vi "G#Installer.vi"() -> ()   [LabVIEW 2012, in "G#Installer.lvlib"]
uses:
  Install-support/G#Installer.lvlib
  <vilib>/Utility/error.llb/DialogType.ctl
panel:
  in  "Uninstall":bool
  out "Info":string
  in  "Cancel":bool
  out "License":string="G# Framework\n\nCopyright (c) 2010-2016, AddQ Consulting <http://www.addq.se>\n\nAll rights reserved.\n\n3-clause license (\"New BSD License\" or \"Modified BSD License\")\n(http://en.wikipedia.org/wiki/BSD_license#3-clause_license_.28.22New_BSD_License.22_or_.22Modified_BSD_License.22.29)\n--------------------------------------------------------------------\nBSD LICENSE  (http://www.opensource.org/licenses/bsd-license.php).\n\nRedistribution and use in source and binary forms, with or without modification, are permitted provided that the following conditions are met:\n\nRedistributions of source code must retain the above copyright notice, this list of conditions and the following disclaimer. Redistributions in binary form must reproduce the above copyright notice, this list of conditions and the following disclaimer in the documentation and/or other materials provided with the distribution. Neither the name of AddQ nor the names of its contributors may be used to endorse or promote products derived from this software without specific prior written permission.\n\nTHIS SOFTWARE IS PROVIDED BY THE COPYRIGHT HOLDERS AND CONTRIBUTORS \"AS IS\" AND ANY EXPRESS OR IMPLIED WARRANTIES, INCLUDING, BUT NOT LIMITED TO, THE IMPLIED WARRANTIES OF MERCHANTABILITY AND FITNESS FOR A PARTICULAR PURPOSE ARE DISCLAIMED. IN NO EVENT SHALL THE COPYRIGHT HOLDER OR CONTRIBUTORS BE LIABLE FOR ANY DIRECT, INDIRECT, INCIDENTAL, SPECIAL, EXEMPLARY, OR CONSEQUENTIAL DAMAGES (INCLUDING, BUT NOT LIMITED TO, PROCUREMENT OF SUBSTITUTE GOODS OR SERVICES; LOSS OF USE, DATA, OR PROFITS; OR BUSINESS INTERRUPTION) HOWEVER CAUSED AND ON ANY THEORY OF LIABILITY, WHETHER IN CONTRACT, STRICT LIABILITY, OR TORT (INCLUDING NEGLIGENCE OR OTHERWISE) ARISING IN ANY WAY OUT OF THE USE OF THIS SOFTWARE, EVEN IF ADVISED OF THE POSSIBILITY OF SUCH DAMAGE."
  in  "Install":bool
  # "G# Installer"
  # "1. Installs G# root classes and debugger in vi.lib/addons.\n2. Installs G# IDE in resources/AddQ/G#IDE.\n3. Installs G# examples, menues and help."
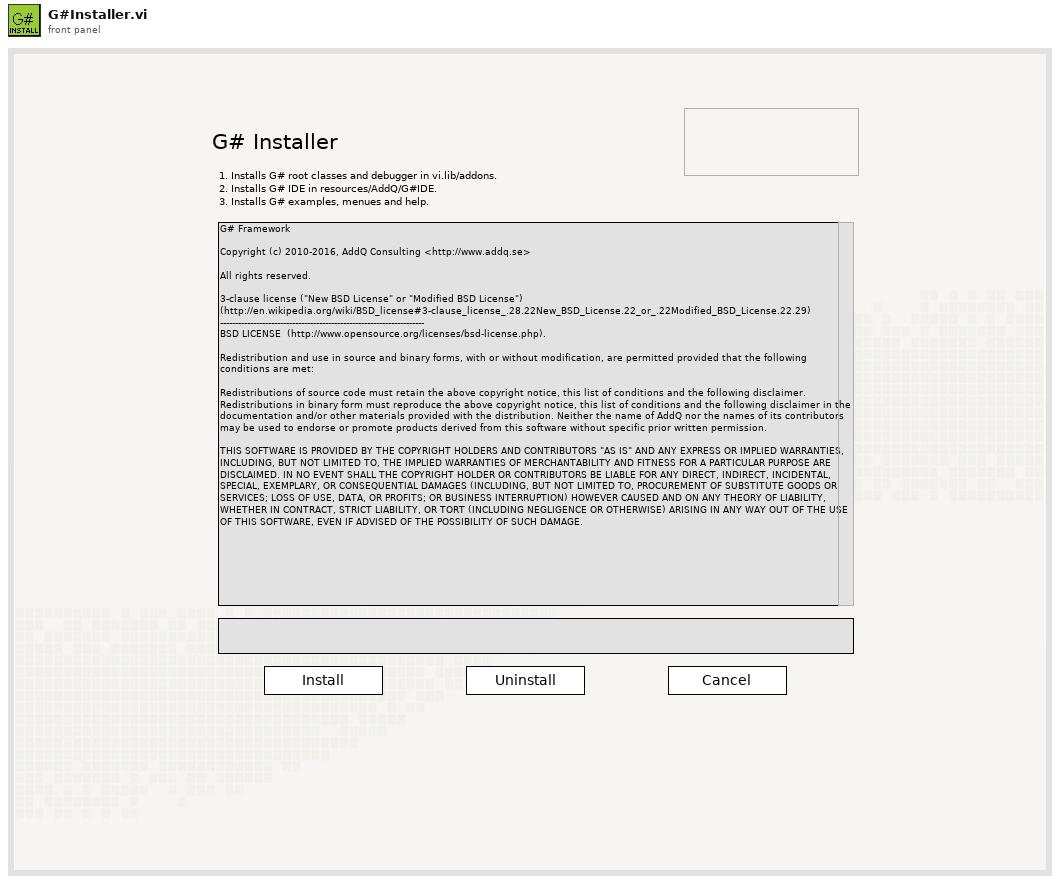
[diagram p1: front panel]
types:
  T1 = enum8{"Enabled", "Disabled", "Disabled and Grayed Out"}
  T2 = typedef "DialogType.ctl" = u16
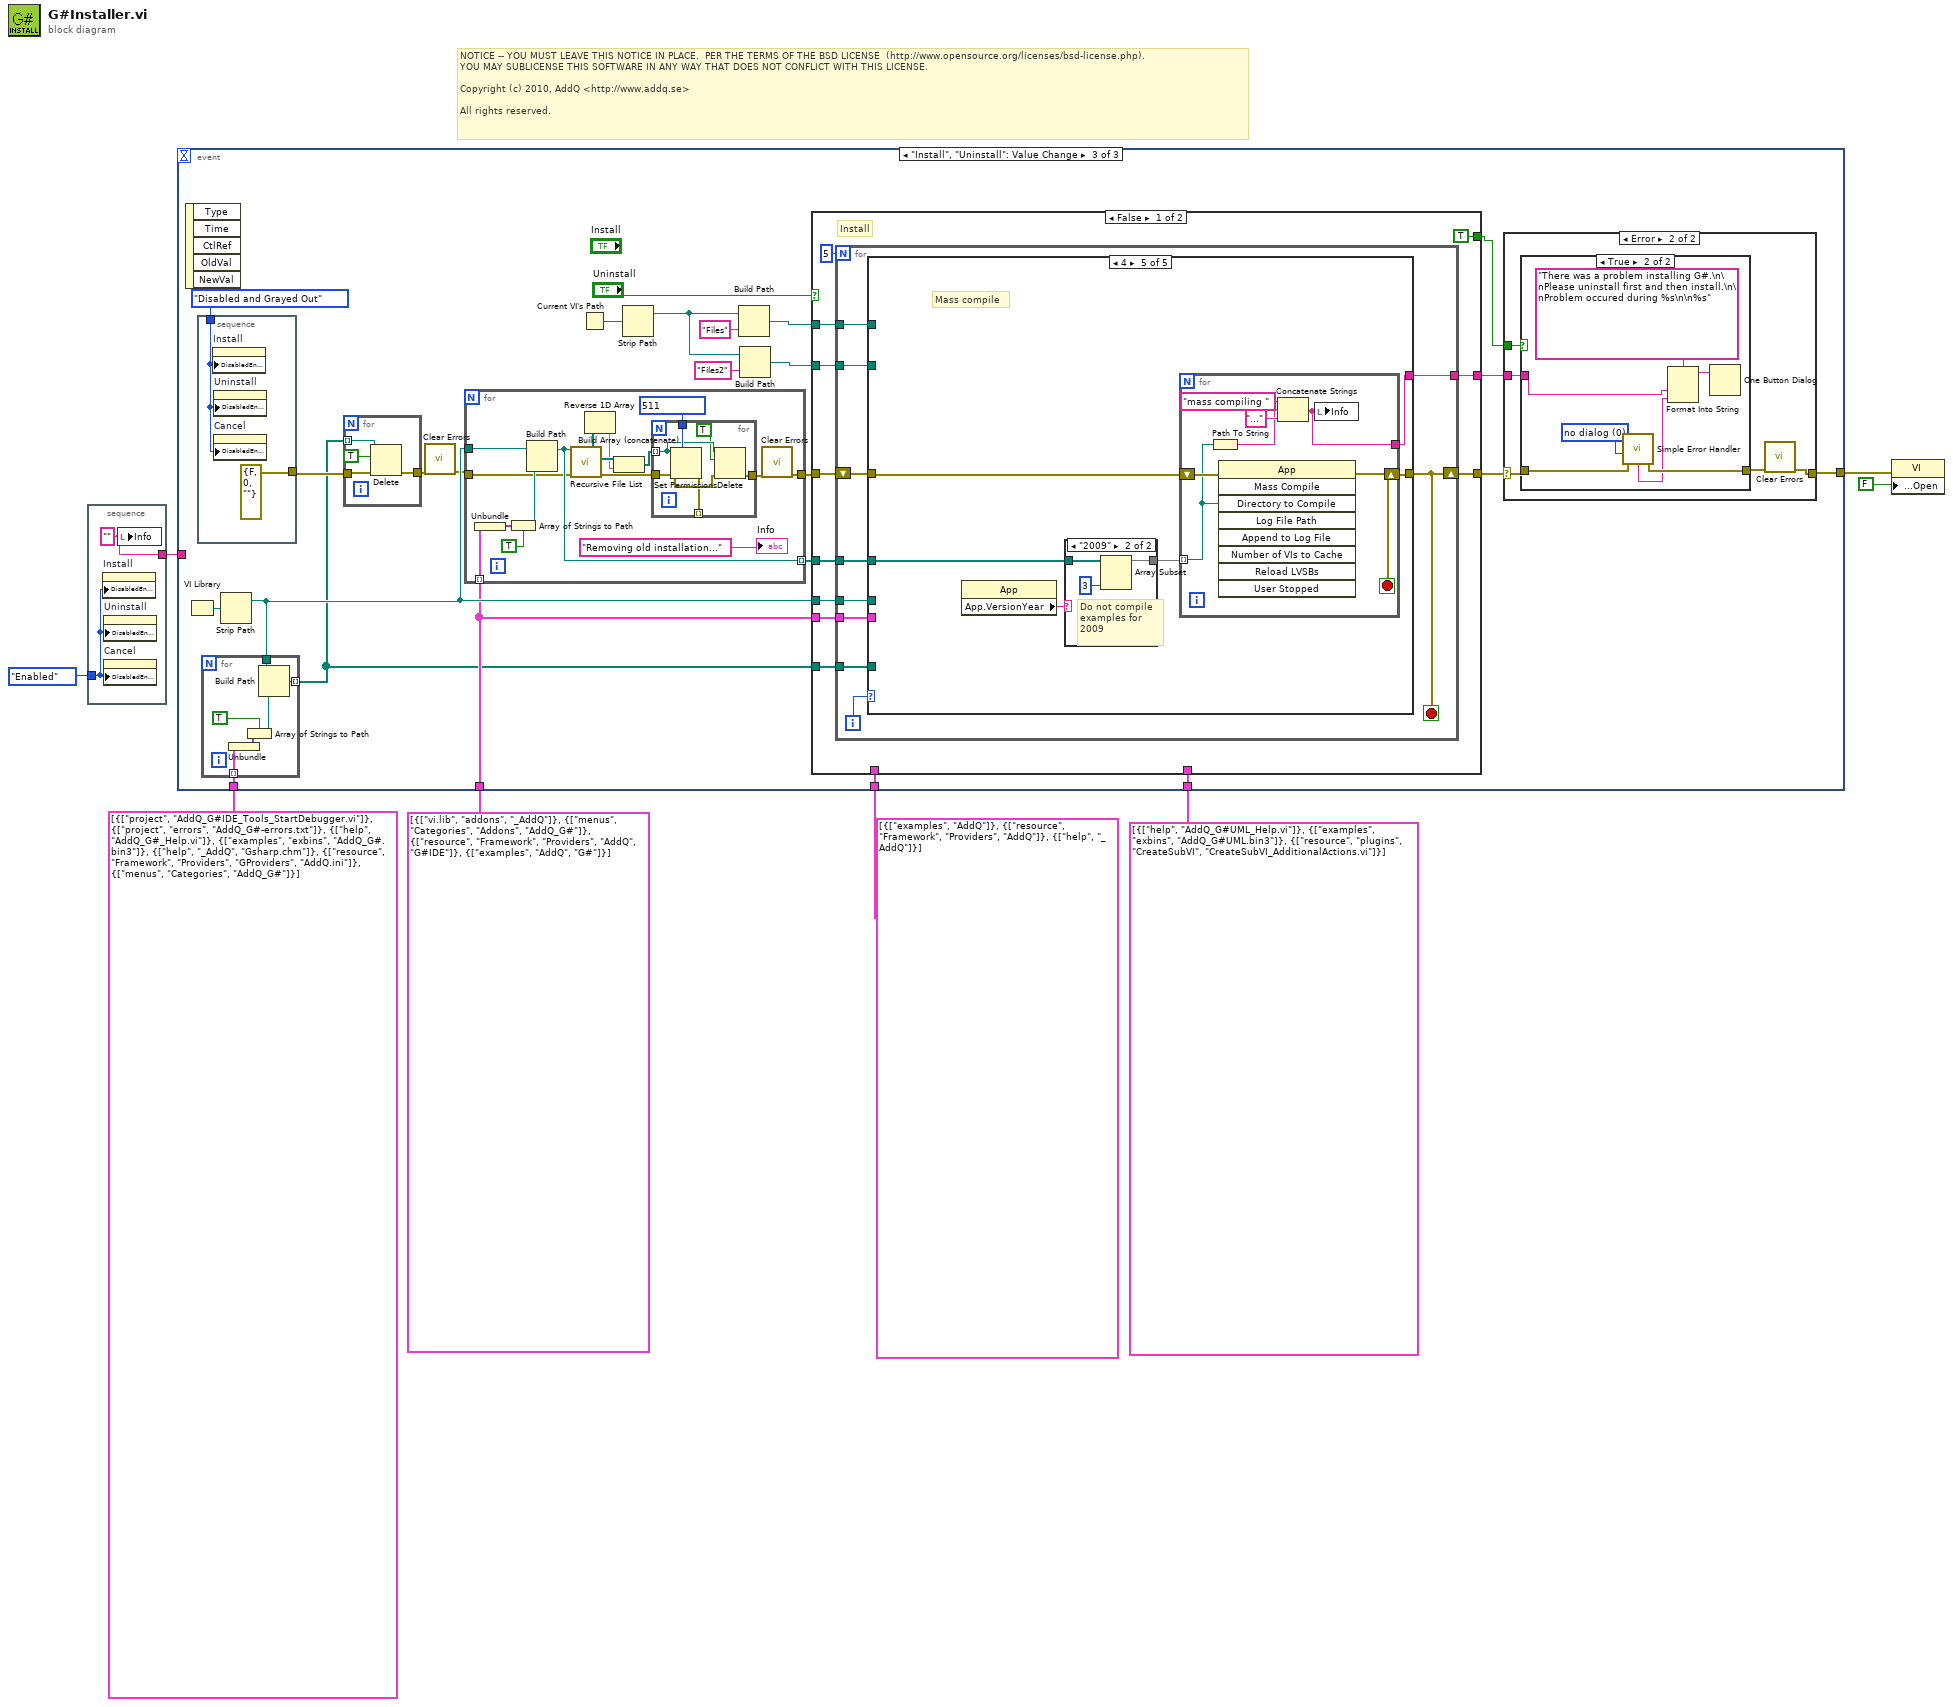
[diagram p0: block diagram]
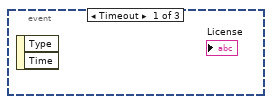
[diagram p2: hidden frame]
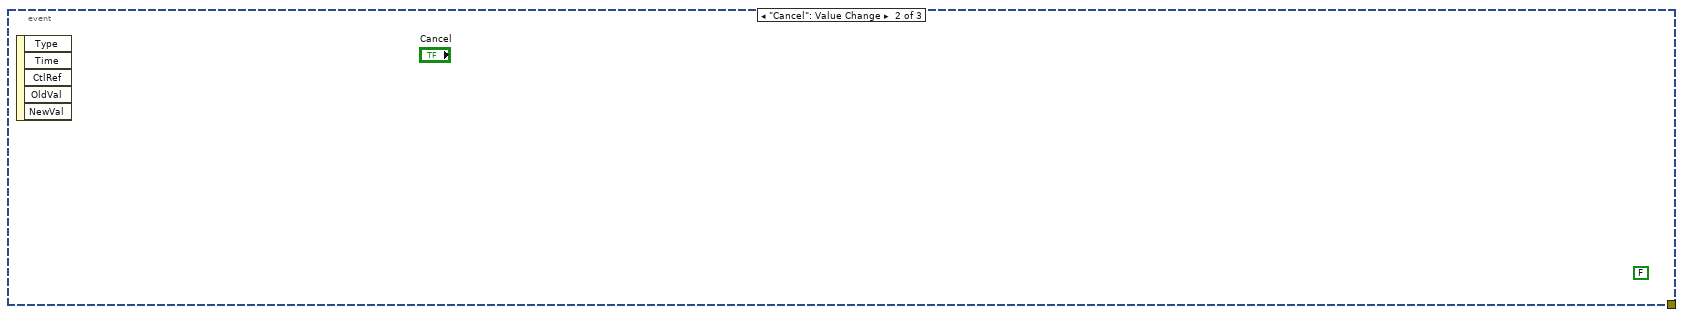
[diagram p3: hidden frame]
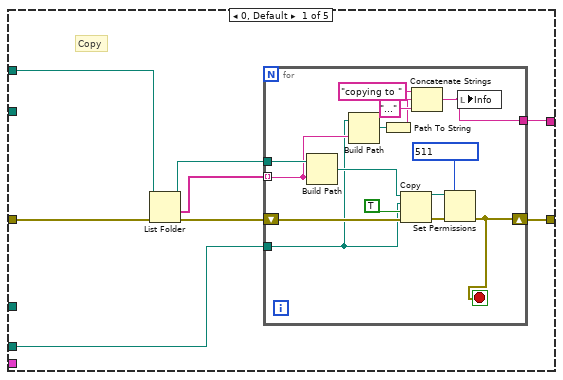
[diagram p4: hidden frame]
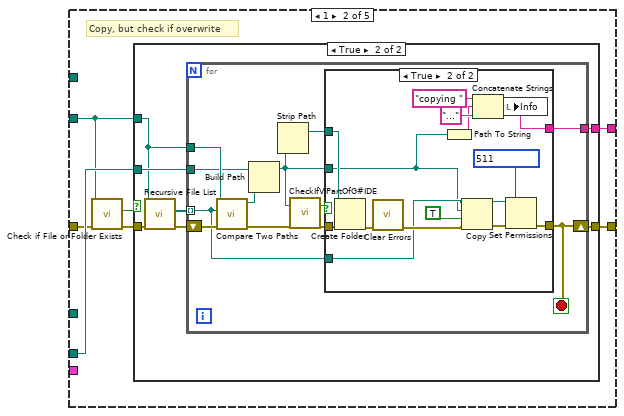
[diagram p5: hidden frame]
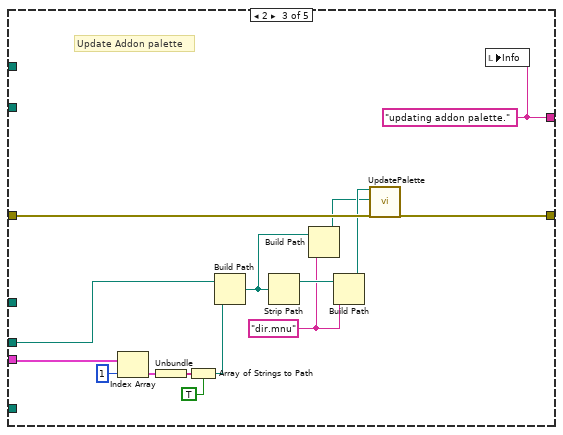
[diagram p8: hidden frame]
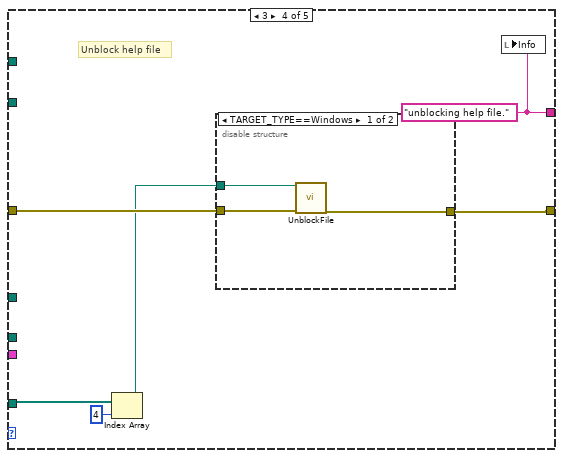
[diagram p9: hidden frame]
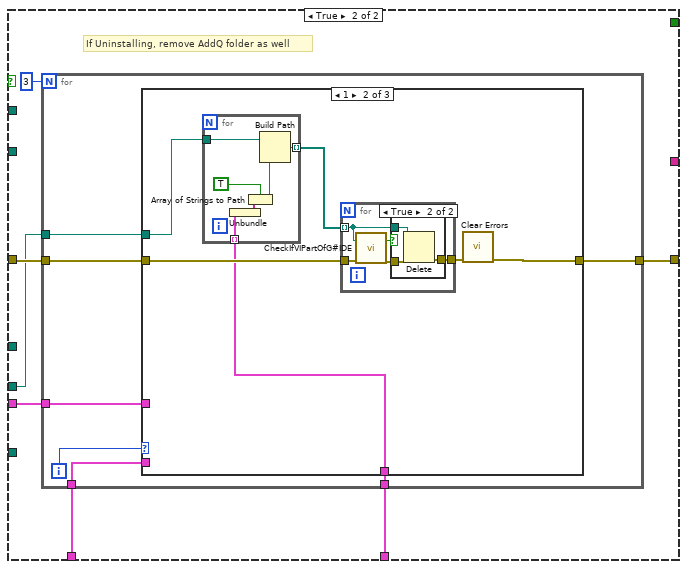
[diagram p12: hidden frame]
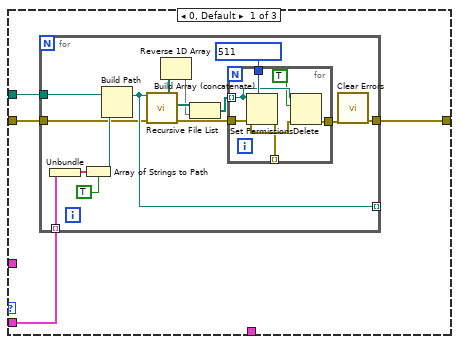
[diagram p13: hidden frame]
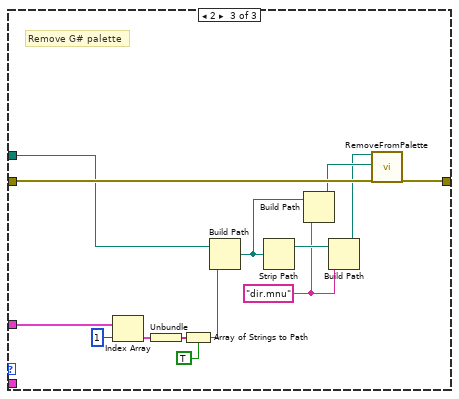
[diagram p15: hidden frame]
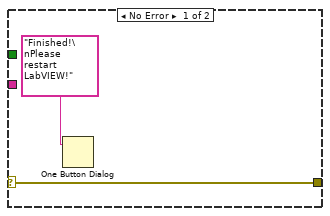
[diagram p16: hidden frame]
diagram:
  # "NOTICE -- YOU MUST LEAVE THIS NOTICE IN PLACE.  PER THE TERMS OF THE BSD LICENSE  (http://www.opensource.org/licenses/bsd-license.php).\nYOU MAY SUBLICENSE THIS SOFTWARE IN ANY WAY THAT DOES NOT CONFLICT WITH THIS LICENSE.\n\nCopyright (c) 2010, AddQ <http://www.addq.se>\n\nAll rights reserved."
  n1 = stacked-sequence {
    tunnel: [w10] -> w8
    tunnel: T1."Enabled" ("Disabled") -> [w9]
    frame #0 {
      w10 = "" ("Info")
      n2 = property on="Install" class="Bool"("DisabledEnum"=w9) -> ()  [unwired: 2 in, 2 out]
      n3 = property on="Uninstall" class="Bool"("DisabledEnum"=w9) -> ()  [unwired: 2 in, 2 out]
      n4 = property on="Cancel" class="Bool"("DisabledEnum"=w9) -> ()  [unwired: 2 in, 2 out]
      n5 = local write "Info"(w10) -> ()
    }
  }
  n6 = event shown="[2] \"Install\", \"Uninstall\": Value Change" {
    selector: _ -> [_ _ _]
    dyn-events: _ -> [_ _ _]
    timeout: _ -> [_ _ _]
    tunnel: w8 -> [_ _ _]
    tunnel: [_ _ w31] -> w1
    tunnel: cluster{string[]}[] [{["vi.lib", "addons", "_AddQ"]}, {["menus", "Categories", "Addons", "AddQ_G#"]}, {["resource", "Framework", "Providers", "AddQ", "G#IDE"]}, {["examples", "AddQ", "G#"]}] -> [_ _ w14]
    tunnel: cluster{string[]}[] [{["project", "AddQ_G#IDE_Tools_StartDebugger.vi"]}, {["project", "errors", "AddQ_G#-errors.txt"]}, {["help", "AddQ_G#_Help.vi"]}, {["examples", "exbins", "AddQ_G#.bin3"]}, {["help", "_AddQ", "Gsharp.chm"]}, {["resource", "Framework", "Providers", "GProviders", "AddQ.ini"]}, {["menus", "Categories", "AddQ_G#"]}] -> [_ _ w26]
    tunnel: cluster{string[]}[] [{["examples", "AddQ"]}, {["resource", "Framework", "Providers", "AddQ"]}, {["help", "_AddQ"]}] -> [_ _ w25]
    tunnel: cluster{string[]}[] [{["help", "AddQ_G#UML_Help.vi"]}, {["examples", "exbins", "AddQ_G#UML.bin3"]}, {["resource", "plugins", "CreateSubVI", "CreateSubVI_AdditionalActions.vi"]}] -> [_ _ w24]
    event Timeout {
      n7 = event-data() -> ()  [unwired: 1 in, 2 out]
    }
    event "Cancel": Value Change {
      (unwired) FALSE ("true")
      n8 = event-data() -> ()  [unwired: 1 in, 5 out]
    }
    event "Install", "Uninstall": Value Change {
      n9 = event-data() -> ()  [unwired: 1 in, 5 out]
      n10 = VI Library() -> (path=w32:path)
      n11 = stacked-sequence {
        tunnel: T1."Disabled and Grayed Out" ("Disabled") -> [w36]
        tunnel: [errorcluster {"status"=FALSE, "code"=0, "source"=""} ("error out")] -> w17
        frame #0 {
          n12 = property on="Install" class="Bool"("DisabledEnum"=w36) -> ()  [unwired: 2 in, 2 out]
          n13 = property on="Uninstall" class="Bool"("DisabledEnum"=w36) -> ()  [unwired: 2 in, 2 out]
          n14 = property on="Cancel" class="Bool"("DisabledEnum"=w36) -> ()  [unwired: 2 in, 2 out]
        }
      }
      n15 = Strip Path(path=w32) -> (stripped path=w22:path)  [unwired: 1 out]
      n16 = for {
        tunnel: w22 -> [w42]
        tunnel: [w41] -> w13 mode=indexing
        tunnel: w26 -> [w40] mode=indexing
        n17 = Unbundle(w40) -> (w38:string[])
        n18 = Array of Strings to Path(0:w38, 1:TRUE ("relative")) -> (2:w37:path)
        n19 = Build Path(base path=w42, name or relative path=w37) -> (appended path=w41:path)
      }
      n20 = for {
        tunnel: [w46] -> w27
        tunnel: w17 -> [w44]
        tunnel: w13 -> [w45] mode=indexing
        n21 = Delete(path (use dialog)=w45, entire hierarchy (F)=TRUE, error in=w44) -> (error out=w46:errorcluster)  [unwired: 2 in, 2 out]
      }
      n22 = call <vilib>:"Clear Errors.vi"("error in (no error)"=w27) -> ("error out"=w16:errorcluster)  [unwired: 6 in]
      n23 = for {
        tunnel: w22 -> [w264]
        tunnel: [w263] -> w15
        tunnel: [w252] -> w28 mode=indexing
        tunnel: w14 -> [w256] mode=indexing
        tunnel: w16 -> [w250]
        n24 = Unbundle(w256) -> (w255:string[])
        n25 = Array of Strings to Path(0:w255, 1:TRUE ("relative")) -> (2:w254:path)
        n26 = Build Path(base path=w264, name or relative path=w254) -> (appended path=w252:path)
        n27 = call <vilib>:"Recursive File List.vi"("error in (no error)"=w250, "Folder Path"=w252) -> ("error out"=w262:errorcluster, "All Files in Dir"=w260:path[], "All Folders"=w258:path[])  [unwired: 5 in, 2 out]
        n28 = Reverse 1D Array(array=w258) -> (reversed array=w257:path[])
        n29 = Build Array (concatenate)(w260, w257) -> (w259:path[])
        n30 = for {
          tunnel: i16 511 ("permissions") -> [w271]
          tunnel: w262 -> [w269]
          tunnel: w259 -> [w268] mode=indexing
          tunnel: [w270] -> w261
          tunnel: [w267] -> _ mode=indexing
          n31 = Set Permissions(7:w271, 8:w269, 11:w268) -> (0:w267:errorcluster)  [unwired: 2 in, 1 out]
          n32 = Delete(path (use dialog)=w268, entire hierarchy (F)=TRUE, error in=w269) -> (error out=w270:errorcluster)  [unwired: 2 in, 2 out]
        }
        n33 = call <vilib>:"Clear Errors.vi"("error in (no error)"=w261) -> ("error out"=w263:errorcluster)  [unwired: 6 in]
        "Info" <- "Removing old installation..." ("string")
      }
      n34 = Current VI's Path() -> (path=w34:path)
      n35 = Strip Path(path=w34) -> (stripped path=w21:path)  [unwired: 1 out]
      n36 = Build Path(base path=w21, name or relative path="Files") -> (appended path=w19:path)
      n37 = Build Path(base path=w21, name or relative path="Files2") -> (appended path=w18:path)
      n38 = case shown="False" "Uninstall" {
        tunnel: w19 -> [w57 _]
        tunnel: w22 -> [w56 w180]
        tunnel: [w53 w178] -> w30
        tunnel: w28 -> [w52 _]
        tunnel: w15 -> [w55 w182]
        tunnel: w25 -> [_ w181]
        tunnel: w24 -> [_ w177]
        tunnel: w18 -> [w51 _]
        tunnel: w14 -> [w50 w176]
        tunnel: w13 -> [w49 _]
        tunnel: [w48 _] -> w12
        tunnel: [TRUE ("Install") _] -> w11
        frame False {
          # "Install"
          n39 = for {
            N: 5 -> [_]
            tunnel: w57 -> [w67]
            tunnel: w56 -> [w66]
            shift-right: [w58] -> w53
            shift-left: w55 -> [w65]
            tunnel: w52 -> [w63]
            tunnel: w51 -> [w62]
            tunnel: w50 -> [w61]
            tunnel: w49 -> [w60]
            tunnel: [w59] -> w48
            i -> [w64]
            stop <- w58 stop-if-true
            n40 = case shown="4" w64 {
              tunnel: w67 -> [w75 _ _ _ _]
              tunnel: w66 -> [w74 w97 w141 _ _]
              tunnel: w65 -> [w73 w95 w148 w154 w162]
              tunnel: [w72 w96 w135 w150 w164] -> w58
              tunnel: w63 -> [_ _ _ _ w161]
              tunnel: w62 -> [_ w93 _ _ _]
              tunnel: w61 -> [_ _ w147 _ _]
              tunnel: w60 -> [_ _ _ w153 _]
              tunnel: [w68 w91 w134 w149 w159] -> w59
              frame 0, Default {
                # "Copy"
                n41 = List Folder(path=w75, error in=w73) -> (path out=w71:path, folder names=w69:string[], error out=w70:errorcluster)  [unwired: 2 in, 1 out]
                n42 = for {
                  tunnel: w74 -> [w78]
                  tunnel: w69 -> [w79] mode=indexing
                  tunnel: w71 -> [w89]
                  shift-right: [w77] -> w72
                  shift-left: w70 -> [w86]
                  tunnel: [w76] -> w68
                  stop <- w77 stop-if-true
                  n43 = Build Path(base path=w89, name or relative path=w79) -> (appended path=w82:path)
                  n44 = Build Path(base path=w78, name or relative path=w79) -> (appended path=w80:path)
                  n45 = Path To String(path=w80) -> (string=w81:string)
                  n46 = Copy(8:w86, 9:TRUE ("overwrite (F)"), 10:w78, 11:w82) -> (0:w85:errorcluster, 3:w84:path)  [unwired: 1 in, 1 out]
                  n47 = Concatenate Strings("copying to " ("string"), w81, "..." ("string")) -> (w76:string)
                  n48 = Set Permissions(7:i16 511 ("permissions"), 8:w85, 11:w84) -> (0:w77:errorcluster)  [unwired: 2 in, 1 out]
                  n49 = local write "Info"(w76) -> ()
                }
              }
              frame 1 {
                # "Copy, but check if overwrite"
                n50 = call <vilib>:"Check if File or Folder Exists.vi"("error in (no error)"=w95, "path"=w93) -> ("error out"=w94:errorcluster, "file or folder exists?"=w92:bool)  [unwired: 7 in, 1 out]
                n51 = case shown="True" w92 {
                  tunnel: w97 -> [_ w105]
                  tunnel: [w98 w104] -> w96
                  tunnel: w94 -> [w98 w101]
                  tunnel: w93 -> [_ w100]
                  tunnel: [_ w99] -> w91
                  frame False {
                  }
                  frame True {
                    n52 = call <vilib>:"Recursive File List.vi"("error in (no error)"=w101, "Folder Path"=w100) -> ("error out"=w103:errorcluster, "All Files in Dir"=w102:path[])  [unwired: 5 in, 3 out]
                    n53 = for {
                      tunnel: w105 -> [w112]
                      tunnel: w102 -> [w108] mode=indexing
                      shift-right: [w106] -> w104
                      shift-left: w103 -> [w116]
                      tunnel: w100 -> [w114]
                      tunnel: [w107] -> w99
                      stop <- w106 stop-if-true
                      n54 = call <vilib>:"Compare Two Paths.vi"("error in (no error)"=w116, "Path 2"=w108, "Path 1"=w114) -> ("error out"=w115:errorcluster, "Relative Path from 1 to 2"=w113:path)  [unwired: 5 in, 2 out]
                      n55 = Build Path(base path=w112, name or relative path=w113) -> (appended path=w111:path)
                      n56 = Strip Path(path=w111) -> (stripped path=w109:path)  [unwired: 1 out]
                      n57 = call "CheckIfVIPartOfG#IDE.vi"("Path"=w111, "error in (no error)"=w115) -> ("PartOfG#IDE?"=w110:bool, "error out"=w117:errorcluster)  [unwired: 16 in]
                      n58 = case shown="True" w110 {
                        tunnel: [w118 w127] -> w106
                        tunnel: w117 -> [w118 w126]
                        tunnel: w111 -> [_ w121]
                        tunnel: w109 -> [_ w123]
                        tunnel: w108 -> [_ w122]
                        tunnel: [_ w119] -> w107
                        frame False {
                          # "There already exist an unknown file,\ndon't overwrite."
                        }
                        frame True {
                          n59 = Create Folder(path (use dialog)=w123, error in=w126) -> (error out=w125:errorcluster)  [unwired: 1 in, 2 out]
                          n60 = call <vilib>:"Clear Errors.vi"("error in (no error)"=w125) -> ("error out"=w124:errorcluster)  [unwired: 6 in]
                          n61 = Path To String(path=w121) -> (string=w120:string)
                          n62 = Copy(8:w124, 9:TRUE ("overwrite (F)"), 10:w121, 11:w122) -> (0:w130:errorcluster, 3:w129:path)  [unwired: 1 in, 1 out]
                          n63 = Concatenate Strings("copying " ("string"), w120, "..." ("string")) -> (w119:string)
                          n64 = local write "Info"(w119) -> ()
                          n65 = Set Permissions(7:i16 511 ("permissions"), 8:w130, 11:w129) -> (0:w127:errorcluster)  [unwired: 2 in, 1 out]
                        }
                      }
                    }
                  }
                }
              }
              frame 2 {
                w134 = "updating addon palette."
                w137 = "dir.mnu" ("name or relative path")
                # "Update Addon palette"
                n66 = Index Array(array=w147, index=1) -> (element=w145:cluster{string[]})
                n67 = Unbundle(w145) -> (w142:string[])
                n68 = Array of Strings to Path(0:w142, 1:TRUE ("relative")) -> (2:w143:path)
                n69 = Build Path(base path=w141, name or relative path=w143) -> (appended path=w138:path)
                n70 = Strip Path(path=w138) -> (stripped path=w140:path)  [unwired: 1 out]
                n71 = Build Path(base path=w138, name or relative path=w137) -> (appended path=w136:path)
                n72 = Build Path(base path=w140, name or relative path=w137) -> (appended path=w139:path)
                n73 = call "UpdatePalette.vi"("palette path"=w139, "SubmenuPath"=w136, "error in (no error)"=w148) -> ("error out"=w135:errorcluster)  [unwired: 16 in]
                n74 = local write "Info"(w134) -> ()
              }
              frame 3 {
                w149 = "unblocking help file."
                # "Unblock help file"
                n75 = Index Array(array=w153, index=4) -> (element=w151:path)
                n76 = disable-structure shown="TARGET_TYPE==Windows" {
                  disable-tunnel: w154 -> [w157 w158]
                  disable-tunnel: w151 -> [w156 _]
                  disable-tunnel: [w155 w158] -> w150
                  frame condition #0 (active) {
                    n77 = call "UnblockFile.vi"("source path"=w156, "error in (no error)"=w157) -> ("error out"=w155:errorcluster)  [unwired: 17 in]
                  }
                  frame condition #1 {
                  }
                }
                n78 = local write "Info"(w149) -> ()
              }
              frame 4 {
                # "Mass compile"
                n79 = property class="App"() -> ("App.VersionYear"=w163:string)  [unwired: 2 in, 2 out]
                n80 = case shown="\"2009\"" w163 {
                  tunnel: w161 -> [w165 w168]
                  tunnel: [w165 w167] -> w160
                  frame Default {
                  }
                  frame "2009" {
                    # "Do not compile\nexamples for\n2009"
                    n81 = Array Subset(array=w168, length=3) -> (w167:path[])  [unwired: 1 in]
                  }
                }
                n82 = for {
                  shift-right: [w170] -> w164
                  shift-left: w162 -> [w175]
                  tunnel: w160 -> [w172] mode=indexing
                  tunnel: [w169] -> w159
                  stop <- w170 stop-if-true
                  n83 = Path To String(path=w172) -> (string=w171:string)
                  n84 = invoke class="App" method="Mass Compile"(error in=w175, "Directory to Compile"=w172) -> (error out=w170:errorcluster)  [unwired: 7 in, 8 out]
                  n85 = Concatenate Strings("mass compiling " ("string"), w171, "..." ("string")) -> (w169:string)
                  n86 = local write "Info"(w169) -> ()
                }
              }
            }
          }
        }
        frame True {
          # "If Uninstalling, remove AddQ folder as well"
          n87 = for {
            N: 3 -> [_]
            tunnel: w182 -> [w189]
            tunnel: w181 -> [w188]
            tunnel: w180 -> [w187]
            tunnel: [w185] -> w178
            tunnel: w177 -> [w184]
            tunnel: w176 -> [w183]
            i -> [w186]
            n88 = case shown="1" w186 {
              tunnel: w189 -> [w193 w218 w241]
              tunnel: w188 -> [w192 _ _]
              tunnel: w187 -> [w191 w216 w236]
              tunnel: [w190 w217 w238] -> w185
              tunnel: w184 -> [_ w215 _]
              tunnel: w183 -> [_ _ w237]
              frame 0, Default {
                n89 = for {
                  tunnel: w191 -> [w207]
                  tunnel: [w206] -> w190
                  tunnel: [w205] -> _ mode=indexing
                  tunnel: w192 -> [w198] mode=indexing
                  tunnel: w193 -> [w194]
                  n90 = Unbundle(w198) -> (w197:string[])
                  n91 = Array of Strings to Path(0:w197, 1:TRUE ("relative")) -> (2:w196:path)
                  n92 = Build Path(base path=w207, name or relative path=w196) -> (appended path=w205:path)
                  n93 = call <vilib>:"Recursive File List.vi"("error in (no error)"=w194, "Folder Path"=w205) -> ("error out"=w204:errorcluster, "All Files in Dir"=w202:path[], "All Folders"=w200:path[])  [unwired: 5 in, 2 out]
                  n94 = Reverse 1D Array(array=w200) -> (reversed array=w199:path[])
                  n95 = Build Array (concatenate)(w202, w199) -> (w201:path[])
                  n96 = for {
                    tunnel: i16 511 ("permissions") -> [w214]
                    tunnel: w204 -> [w212]
                    tunnel: w201 -> [w211] mode=indexing
                    tunnel: [w213] -> w203
                    tunnel: [w210] -> _ mode=indexing
                    n97 = Set Permissions(7:w214, 8:w212, 11:w211) -> (0:w210:errorcluster)  [unwired: 2 in, 1 out]
                    n98 = Delete(path (use dialog)=w211, entire hierarchy (F)=TRUE, error in=w212) -> (error out=w213:errorcluster)  [unwired: 2 in, 2 out]
                  }
                  n99 = call <vilib>:"Clear Errors.vi"("error in (no error)"=w203) -> ("error out"=w206:errorcluster)  [unwired: 6 in]
                }
              }
              frame 1 {
                n100 = for {
                  tunnel: [w226] -> w220 mode=indexing
                  tunnel: w215 -> [w225] mode=indexing
                  tunnel: w216 -> [w221]
                  n101 = Unbundle(w225) -> (w223:string[])
                  n102 = Array of Strings to Path(0:w223, 1:TRUE ("relative")) -> (2:w222:path)
                  n103 = Build Path(base path=w221, name or relative path=w222) -> (appended path=w226:path)
                }
                n104 = for {
                  tunnel: [w231] -> w219
                  tunnel: w218 -> [w230]
                  tunnel: w220 -> [w228] mode=indexing
                  n105 = call "CheckIfVIPartOfG#IDE.vi"("Path"=w228, "error in (no error)"=w230) -> ("PartOfG#IDE?"=w227:bool, "error out"=w229:errorcluster)  [unwired: 16 in]
                  n106 = case shown="True" w227 {
                    tunnel: [w232 w235] -> w231
                    tunnel: w229 -> [w232 w234]
                    tunnel: w228 -> [_ w233]
                    frame False {
                    }
                    frame True {
                      n107 = Delete(path (use dialog)=w233, error in=w234) -> (error out=w235:errorcluster)  [unwired: 3 in, 2 out]
                    }
                  }
                }
                n108 = call <vilib>:"Clear Errors.vi"("error in (no error)"=w219) -> ("error out"=w217:errorcluster)  [unwired: 6 in]
              }
              frame 2 {
                w242 = "dir.mnu" ("name or relative path")
                # "Remove G# palette"
                n109 = Index Array(array=w237, index=1) -> (element=w248:cluster{string[]})
                n110 = Unbundle(w248) -> (w245:string[])
                n111 = Array of Strings to Path(0:w245, 1:TRUE ("relative")) -> (2:w246:path)
                n112 = Build Path(base path=w236, name or relative path=w246) -> (appended path=w243:path)
                n113 = Strip Path(path=w243) -> (stripped path=w244:path)  [unwired: 1 out]
                n114 = Build Path(base path=w243, name or relative path=w242) -> (appended path=w240:path)
                n115 = Build Path(base path=w244, name or relative path=w242) -> (appended path=w239:path)
                n116 = call "RemoveFromPalette.vi"("palette path"=w239, "SubmenuPath"=w240, "error in (no error)"=w241) -> ("error out"=w238:errorcluster)  [unwired: 16 in]
              }
            }
          }
        }
      }
      n117 = case shown="Error" w30 {
        selector: w30 -> [w273 w278]
        tunnel: [w273 w274] -> w31
        tunnel: w12 -> [_ w276]
        tunnel: w11 -> [_ w277]
        frame No Error {
          n118 = One Button Dialog(message="Finished!\nPlease restart LabVIEW!") -> ()  [unwired: 1 in, 1 out]
        }
        frame Error {
          n119 = case shown="True" w277 {
            tunnel: w278 -> [w279 w283]
            tunnel: [w279 w282] -> w275
            tunnel: w276 -> [_ w280]
            frame False {
            }
            frame True {
              w285 = T2 0 items=["no dialog", "OK message", "continue or stop message", "OK message + warnings", "continue/stop + warnings"] ("type of dialog (OK msg:1)")
              n120 = call <vilib>:"Simple Error Handler.vi"("type of dialog (OK msg:1)"=w285, "error in (no error)"=w283) -> ("error out"=w282:errorcluster, "message"=w281:string)  [unwired: 3 in, 3 out]
              n121 = Format Into String(format string="There was a problem installing G#.\n\nPlease uninstall first and then install.\n\nProblem occured during %s\n\n%s", w280, w281) -> (resulting string=w284:string)  [unwired: 2 in, 1 out]
              n122 = One Button Dialog(message=w284) -> ()  [unwired: 1 in, 1 out]
            }
          }
          n123 = call <vilib>:"Clear Errors.vi"("error in (no error)"=w275) -> ("error out"=w274:errorcluster)  [unwired: 6 in]
        }
      }
    }
  }
  n124 = property class="VI"(error in=w1, "Front Panel.Open"=FALSE ("Front Panel Window:Open")) -> ()  [unwired: 1 in, 2 out]
